vi "Configure Frequency (Center Span).vi"(0 "VISA resource name":refnum<visa-resource-name>, 1 "Auto Frequency Step Size (T: Enable)":bool=TRUE, 2 "Frequency Step Size (7E+8 Hz)":dbl=700000000.0, 5 "Frequency Mode (0: UP)":i32(ring) items=["Up", "Down", "Manually Input"], 7 "Center Frequency (3.5E+9 Hz)":dbl=3500000000.0, 9 "Frequency Span Mode (0: Previous)":i32(ring) items=["Previous", "Full", "Zero", "Manually Input"], 11 "error in (no error)":errorcluster, 12 "Frequency Span (7E+9 Hz)":dbl=7000000000.0) -> (4 "VISA resource name out":refnum<visa-resource-name>, 15 "error out":errorcluster)   [LabVIEW 2022 SP3, in "Agilent N934X Series.lvlib"]
doc: "Configures the frequency range of the spectrum analyzer using the center frequency and the frequency span. If span corresponds to zero Hertz, then the spectrum analyzer operates in time-domain mode. Otherwise, spectrum analyzer operates in frequency-domain mode.\n\n Frequency Start = Center Frequency - Span/2\n Frequency Stop = Center Frequency + Span/2"
uses:
  <instrlib>/Agilent N934X Series/Agilent N934X Series.lvlib
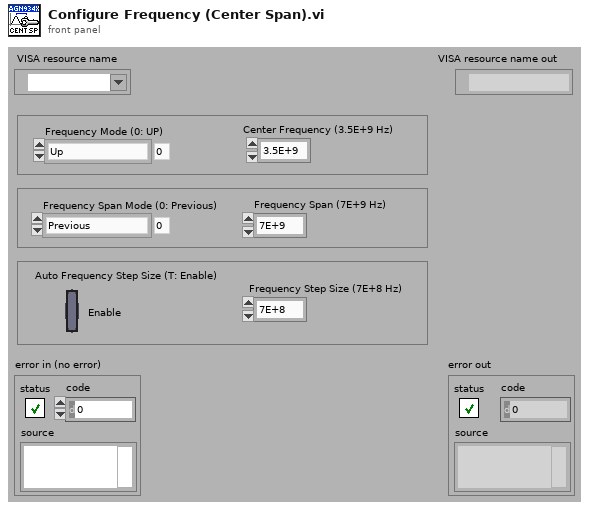
[diagram p1: front panel]
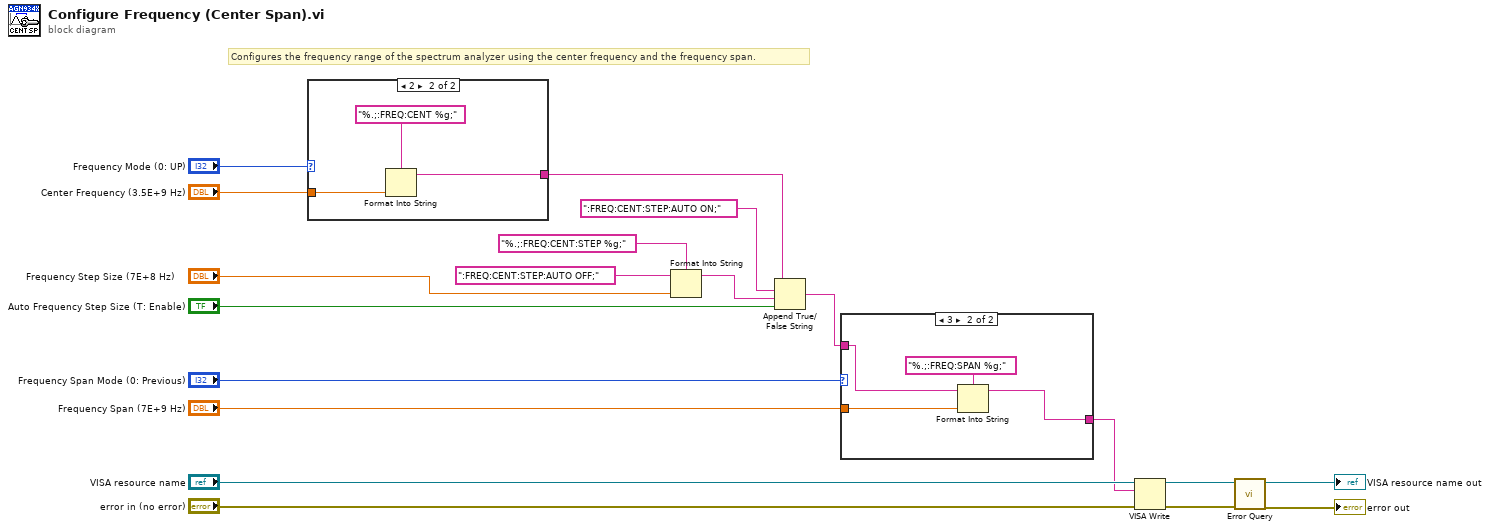
[diagram p0: block diagram]
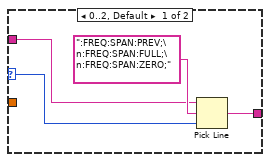
[diagram p2: hidden frame]
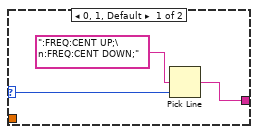
[diagram p3: hidden frame]
diagram:
  # "Configures the frequency range of the spectrum analyzer using the center frequency and the frequency span."
  n1 = case shown="2" "Frequency Mode (0: UP)" {
    selector: "Frequency Mode (0: UP)" -> [w21 _]
    tunnel: "Center Frequency (3.5E+9 Hz)" -> [_ w24]
    tunnel: [w20 w23] -> w10
    frame 0, 1, Default {
      n2 = Pick Line(multi-line string=":FREQ:CENT UP;\n:FREQ:CENT DOWN;", line index=w21) -> (output string=w20:string)  [unwired: 1 in]
    }
    frame 2 {
      n3 = Format Into String(format string="%.;:FREQ:CENT %g;", w24) -> (resulting string=w23:string)  [unwired: 2 in, 1 out]
    }
  }
  n4 = Format Into String(format string="%.;:FREQ:CENT:STEP %g;", initial string=":FREQ:CENT:STEP:AUTO OFF;", "Frequency Step Size (7E+8 Hz)") -> (resulting string=w4:string)  [unwired: 1 in, 1 out]
  n5 = Append True/False String(1:"Auto Frequency Step Size (T: Enable)", 2:w4, 3:":FREQ:CENT:STEP:AUTO ON;", 4:w10) -> (0:w1:string)
  n6 = case shown="3" "Frequency Span Mode (0: Previous)" {
    selector: "Frequency Span Mode (0: Previous)" -> [w29 _]
    tunnel: "Frequency Span (7E+9 Hz)" -> [_ w32]
    tunnel: [w27 w31] -> w2
    tunnel: w1 -> [w26 w30]
    frame 0..2, Default {
      n7 = Pick Line(string ("")=w26, multi-line string=":FREQ:SPAN:PREV;\n:FREQ:SPAN:FULL;\n:FREQ:SPAN:ZERO;", line index=w29) -> (output string=w27:string)
    }
    frame 3 {
      n8 = Format Into String(format string="%.;:FREQ:SPAN %g;", initial string=w30, w32) -> (resulting string=w31:string)  [unwired: 1 in, 1 out]
    }
  }
  n9 = VISA Write(VISA resource name="VISA resource name", write buffer=w2, error in (no error)="error in (no error)") -> (VISA resource name out=w17:refnum<visa-resource-name>, error out=w16:errorcluster)  [unwired: 1 out]
  n10 = call <instrlib>:"Error Query.vi"("error in (no error)"=w16, "VISA resource name"=w17) -> ("error out"=→"error out":errorcluster, "VISA resource name out"=→"VISA resource name out":refnum<visa-resource-name>)  [unwired: 6 in, 2 out]
